vi "Test Run Suite of Test Cases.vi"(8 "error in (no error)":errorcluster, 11 "Test Case In":refnum<class "LUnit Test Suite Tests.lvclass">) -> (0 "error out":errorcluster, 3 "Test Case Out":refnum<class "LUnit Test Suite Tests.lvclass">)   [LabVIEW 2020, in "LUnit Test Suite Tests.lvclass"]
uses:
  LUnit Test Suite Tests.lvclass
  LUnit Test Suite Tests.lvclass/LUnit Test Suite Tests.ctl
  source/LUnit Test Suite.lvclass
  source/Core/Result/Status.ctl
  source/Core/Result/Result.lvlib
  b74e4934-f044-4222-b3dd-fc90e6c1bd4f.vi
  Test Doubles/Test Case Test Double Child/Light Test Case Double.lvclass
  C:/git/astemes-lunit/source/Core/Runnable/Runnable.lvclass
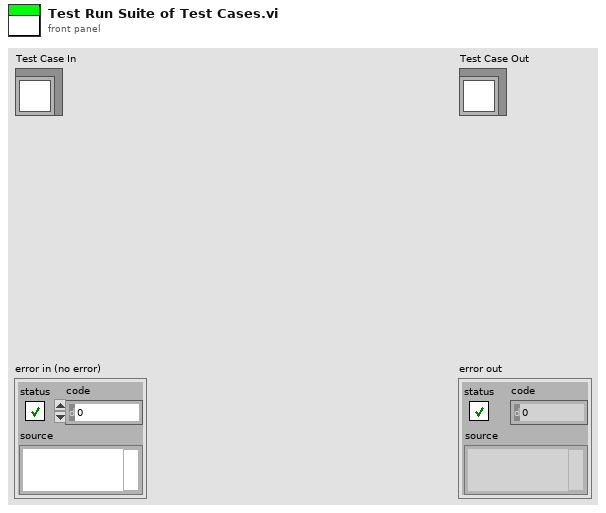
[diagram p1: front panel]
types:
  T1 = typedef "Result.lvlib/Status.ctl" = enum16{"", "Passed", "Failed", "Error", "Skipped", "Setup Error", "Broken", "Teardown Error"}
  T2 = typedef "Result.lvlib/Result.ctl" = cluster{"Name":string, "Description":string, "Status":T1, "Result Type":T3, "Execution Time":dbl, "Data":cluster{"Expected":variant, "Actual":variant, "Delta":variant}}
  T3 = typedef "Result.lvlib/Type.ctl" = enum16{"Test Case", "Test Suite", "Test Run", "Pass", "Fail", "Skip", "Pass if", "Fail if", "Pass if Error", "Fail if Error", "Pass if Equal", "Fail if Equal"}
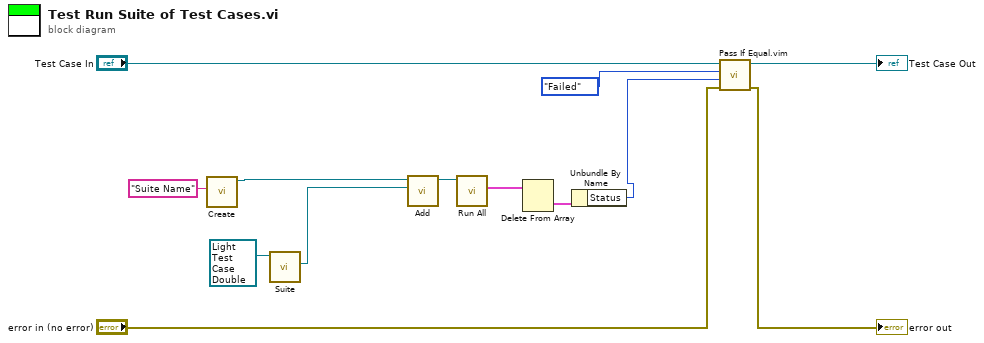
[diagram p0: block diagram]
diagram:
  n1 = call "Create.vi"("Suite Name"="Suite Name") -> ("LUnit Test Suite Out"=w2:refnum<class "LUnit Test Suite.lvclass">)  [unwired: 9 in, 1 out]
  n2 = call-dynamic "Suite.vi"("LUnit Test Case In"=refnum<class "Light Test Case Double.lvclass"> refnum ("LUnit Test Case V2 Test Double.lvclass")) -> ("LUnit Test Suite Out"=w3:refnum<class "LUnit Test Suite.lvclass">)  [unwired: 8 in, 2 out]
  n3 = call "Add.vi"("Runnable"=w3, "LUnit Test Suite In"=w2) -> ("LUnit Test Suite Out"=w9:refnum<class "LUnit Test Suite.lvclass">)  [unwired: 8 in, 1 out]
  n4 = call "Run All.vi"("Runnable In"=w9) -> ("Results"=w8:T2[])  [unwired: 9 in, 1 out]
  n5 = Delete From Array(array=w8) -> (deleted portion=w5:T2)  [unwired: 2 in, 1 out]
  n6 = Unbundle By Name(w5) -> ("Status"=w4:T1)
  n7 = call "Pass If Equal.vim"("error in (no error)"="error in (no error)", "Actual"=w4, "Expected"=Status."Failed" ("Status"), "LUnit Test Case In"="Test Case In") -> ("error out"=→"error out":errorcluster, "LUnit Test Case Out"=→"Test Case Out":refnum<class "LUnit Test Suite Tests.lvclass">)  [unwired: 6 in]
